vi "PSUChargeRelay.vi"(4 "PSU3 Control Panel":T1={"HV Off State"=FALSE, "HV On State"=FALSE, "HV Arm"=FALSE, "HV On"=FALSE, "Charge relay DIO"="DAQ0/port0/line3", "Dump relay DIO"="DAQ0/port0/line4", "HV Arm DIO"="DAQ0/port0/line5", "HV On DIO"="DAQ0/port0/line6", "Bank Voltage [kV]"={0.0, 0.0}, "Vdemand Counter"="Timing1/ctr1", "RevTach Calibration"=path "Z:/Data/Calibration/Reverse Tachometer/PSU2_RevTachCalibration.csv", "Vdemand"=FALSE, "Vmeasure Counter"="Timing1/ctr2", "Tach Calibration"=path "Z:/Data/Calibration/Tachometer/PSU2_TachCalibration.csv", "Vmeasure"=FALSE, "Vdemand [kV]"=0.0, "Charge Relay"=FALSE, "Dump Relay"=FALSE} {"Bank Voltage [kV]" scale=0.01..10.0 scale format="%#_3g"}, 6 "PSU2 Control Panel":T1 {"Bank Voltage [kV]" scale=0.01..10.0 scale format="%#_3g"}, 10 "PSU Relay Variant":T2, 11 "Experiment State in":T3 {"Global Settings"."Initial Background Values"."Cryo temp [K]" format="%#_4g"; "RIO Settings"."Card Settings"."Sample Rate" format="%#_3p"; "Timing Settings"."Timing Channel Settings"."FrontPanelTime" format="%.3p"; "Timing Settings"."Timing Channel Settings"."Pulse width (s)" format="%.3p"; "Timing Settings"."Timing Channel Settings"."Delay (s)" format="%.3p"; "DAQ Settings"."Card Settings"."Global Edge Type" items=["Rising"=10280, "Falling"=10171]; "DAQ Settings"."Card Settings"."Sample Rate" format="%#_3p"}) -> (3 "Experiment State out":T3 {"Global Settings"."Initial Background Values"."Cryo temp [K]" format="%#_4g"; "RIO Settings"."Card Settings"."Sample Rate" format="%#_3p"; "Timing Settings"."Timing Channel Settings"."FrontPanelTime" format="%.3p"; "Timing Settings"."Timing Channel Settings"."Pulse width (s)" format="%.3p"; "Timing Settings"."Timing Channel Settings"."Delay (s)" format="%.3p"; "DAQ Settings"."Card Settings"."Global Edge Type" items=["Rising"=10280, "Falling"=10171]; "DAQ Settings"."Card Settings"."Sample Rate" format="%#_3p"})   [LabVIEW 2014]
uses:
  Controls/PSUPanel-Arming.ctl
  Controls/ExperimentStateCluster.ctl
  Controls/DigitizerSettingsChannelSettings.ctl
  Controls/DigitizerSettingsCardSettingsArray.ctl
  Controls/DigitizerSettingsCardSettings.ctl
  Controls/TimingSettings.ctl
  Controls/TimingCardSettings.ctl
  Controls/TimingChannelSettings.ctl
  Controls/RIOSettingsExperimentStateCluster.ctl
  Controls/RIOChannelSettingsArrayExperimentStateCluster.ctl
  Controls/RIOSettingsChannelSettings.ctl
  Controls/RIOSettingsCardSettingsArray.ctl
  Controls/RIOSettingsCardSettings.ctl
  <vilib>/userdefined/High Color/nirio_resource_hc.ctl
  Controls/RIOData.ctl
  Controls/DIOChannel.ctl
  Controls/Global Settings/GlobalSettings.ctl
  Controls/Global Settings/InitialBackgroundValues.ctl
  Controls/Global Settings/GasPuffing.ctl
  Controls/Global Settings/PSUVoltages.ctl
  Controls/Global Settings/ScopeDetails.ctl
  Controls/Calibrations/Calibrations.ctl
  Controls/Calibrations/CryoTemoCalibration.ctl
  Controls/Calibrations/PSU2TachCalibration.ctl
  Controls/Calibrations/PSU3TachCalibration.ctl
  Controls/TachTasks.ctl
  Controls/PSU2TachometerControls.ctl
  Controls/PSU3TachometerControls.ctl
  Controls/PSU2DIOChannels.ctl
  Controls/PSU3DIOChannels.ctl
  Controls/PSU2ReverseTachometerControls.ctl
  Controls/PSU3ReverseTachometerControls.ctl
  Controls/PSUControlVariant.ctl
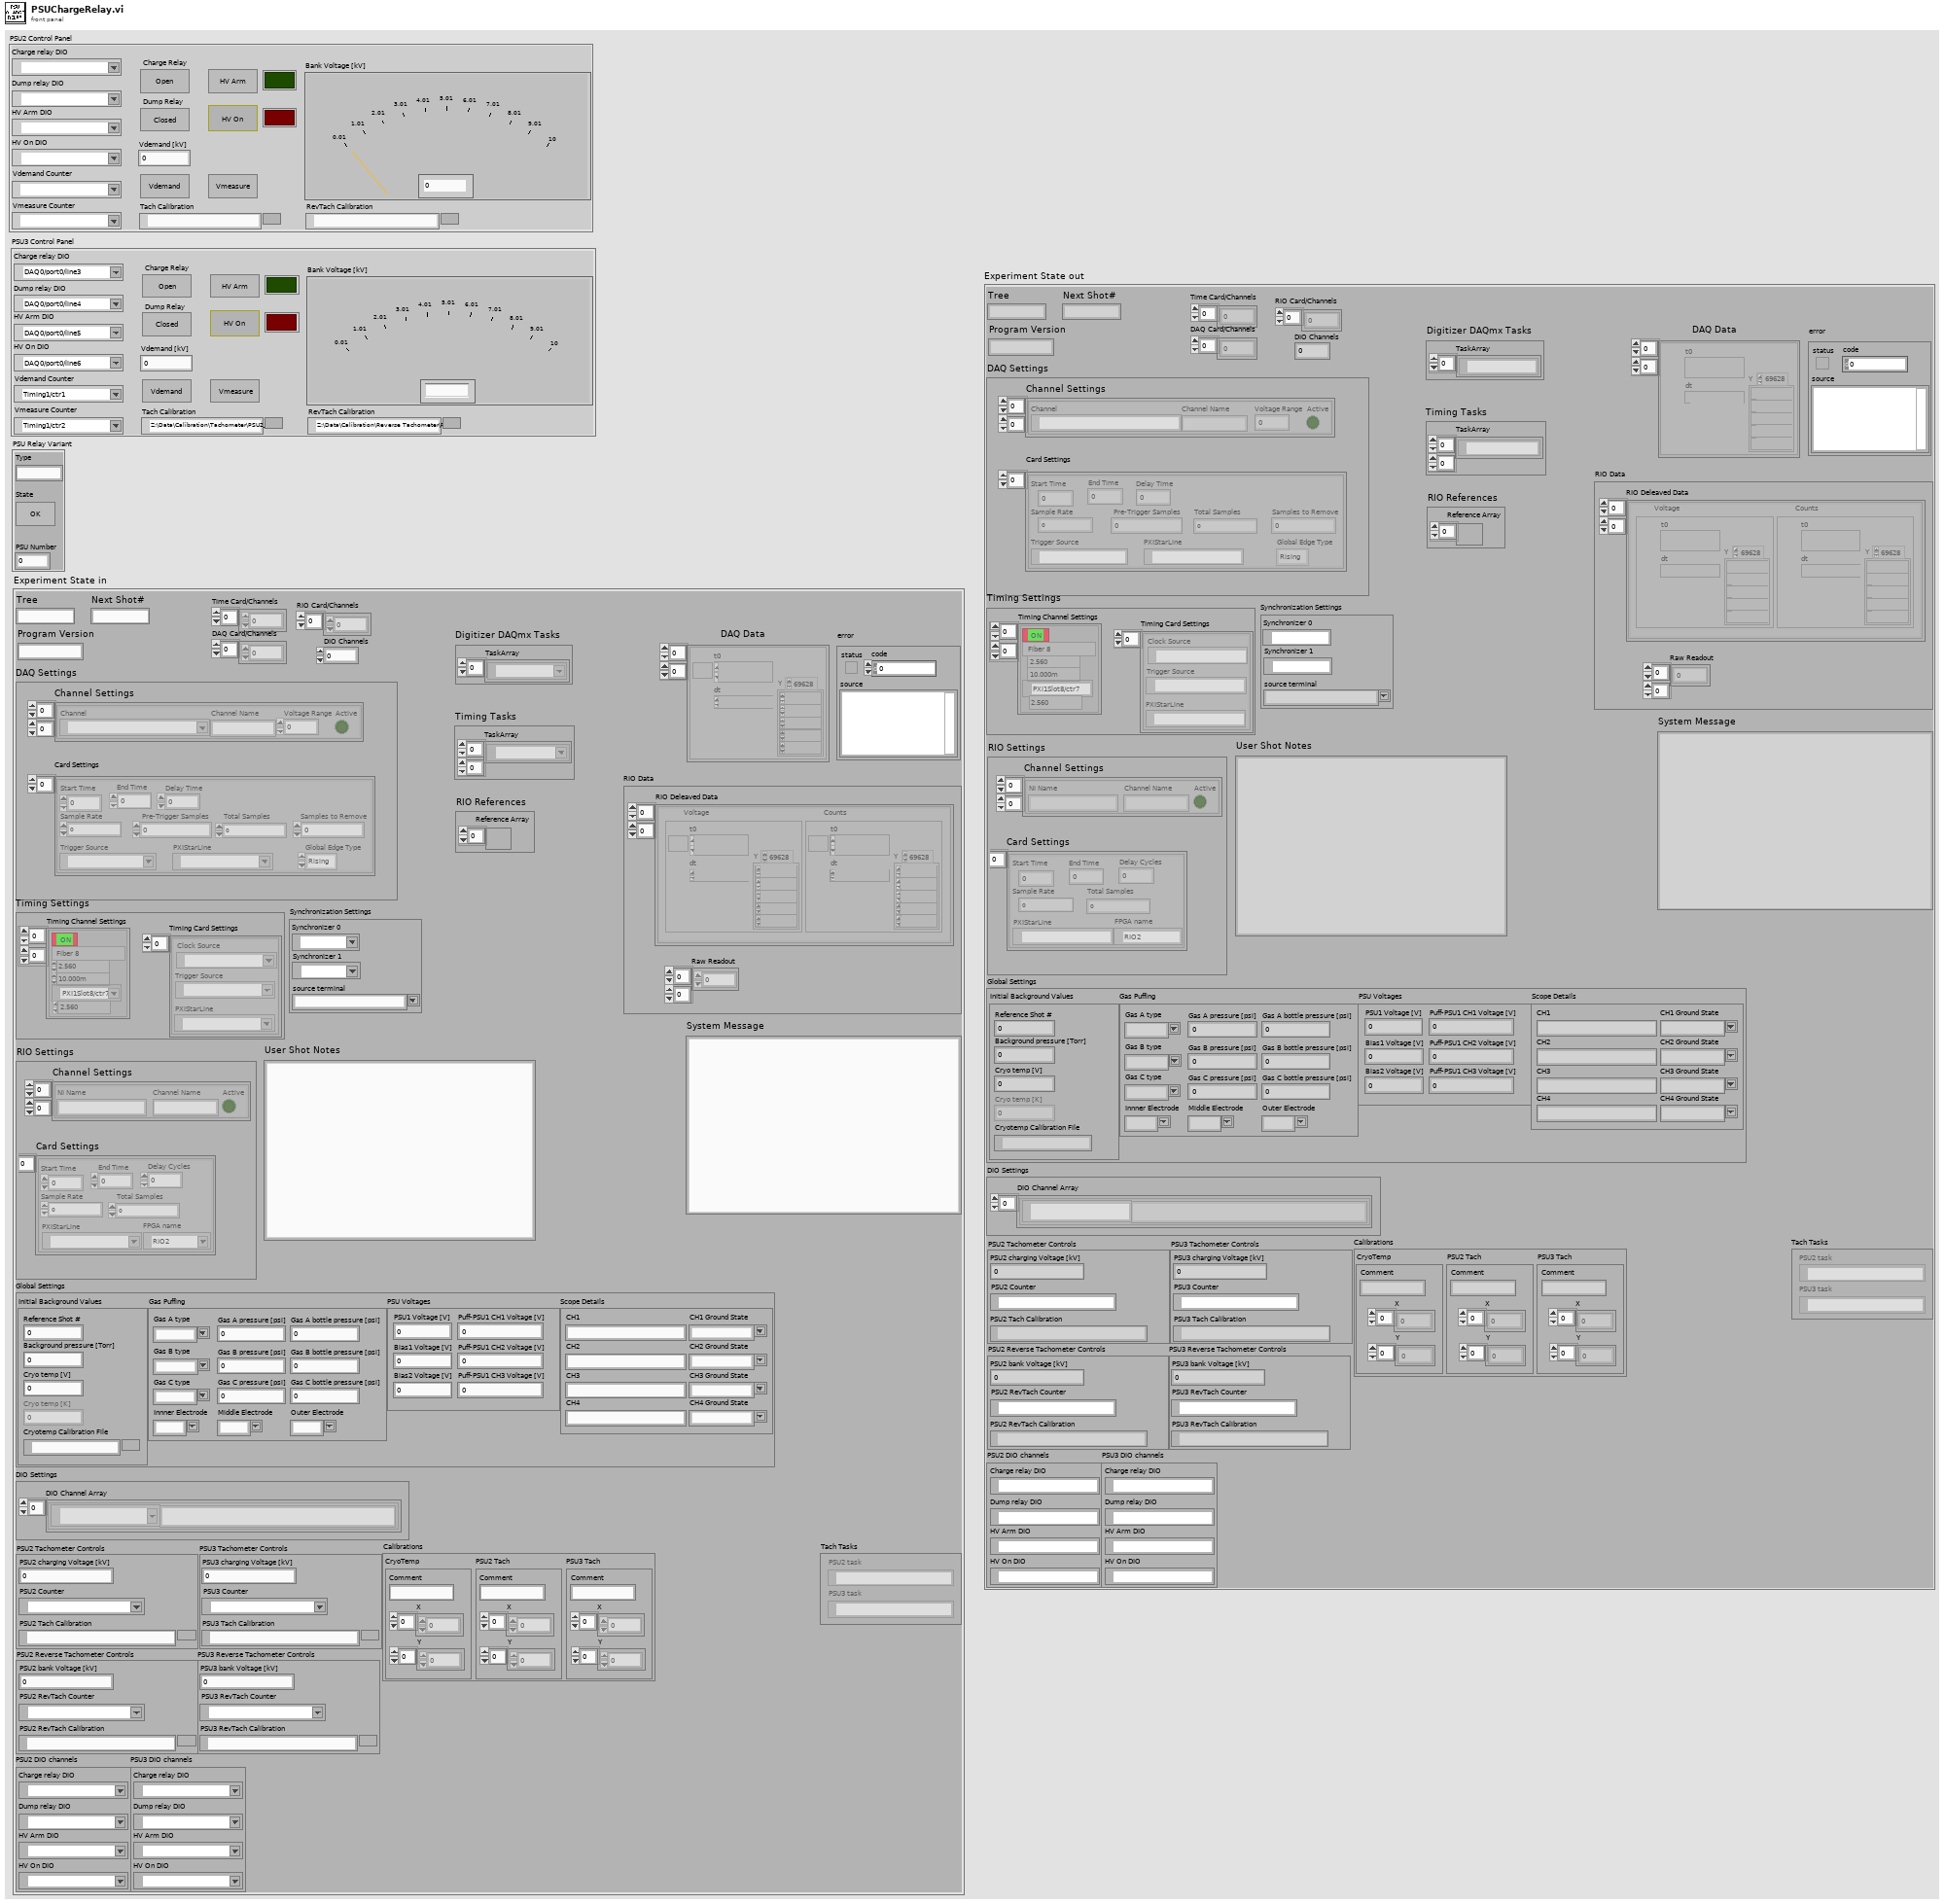
[diagram p1: front panel]
types:
  T1 = typedef "PSUPanel-Arming.ctl" = cluster{"HV Off State":bool, "HV On State":bool, "HV Arm":bool, "HV On":bool, "Charge relay DIO":tag, "Dump relay DIO":tag, "HV Arm DIO":tag, "HV On DIO":tag, "Bank Voltage [kV]":cluster{dbl, dbl}, "Vdemand Counter":tag, "RevTach Calibration":path, "Vdemand":bool, "Vmeasure Counter":tag, "Tach Calibration":path, "Vmeasure":bool, "Vdemand [kV]":dbl, "Charge Relay":bool, "Dump Relay":bool}
  T2 = typedef "PSUControlVariant.ctl" = cluster{"State":bool, "PSU Number":i32, "Type":string}
  T3 = typedef "ExperimentStateCluster.ctl" = cluster{"error":errorcluster, "Digitizer DAQmx Tasks":cluster{"TaskArray":refnum<k21>[]}, "DAQ Settings":cluster{"Channel Settings":T4[][], "Card Settings":T5}, "Synchronization Settings":cluster{"Synchronizer 0":refnum<k15>, "source terminal":string, "Synchronizer 1":refnum<k15>}, "DAQ Data":waveform(dbl)[][], "Next Shot#":string, "System Message":string, "User Shot Notes":string, "Timing Settings":T7, "Timing Tasks":cluster{"TaskArray":refnum<k21>[][]}, "Tree":string, "Time Card/Channels":i32[], "DAQ Card/Channels":i32[], "Program Version":string, "RIO Settings":T10, "RIO References":cluster{"Reference Array":refnum<k20>[]}, "RIO Data":T16, "RIO Card/Channels":i32[], "DIO Channels":i32, "DIO Settings":cluster{"DIO Channel Array":T17[]}, "Global Settings":T18, "Calibrations":T23, "Tach Tasks":T27, "PSU2 Tachometer Controls":T28, "PSU3 Tachometer Controls":T29, "PSU2 DIO channels":T30, "PSU3 DIO channels":T31, "PSU2 Reverse Tachometer Controls":T32, "PSU3 Reverse Tachometer Controls":T33}
  T4 = typedef "DigitizerSettingsChannelSettings.ctl" = cluster{"Channel":tag, "Channel Name":string, "Voltage Range":dbl, "Active":bool}
  T5 = typedef "DigitizerSettingsCardSettingsArray.ctl" = T6[]
  T6 = typedef "DigitizerSettingsCardSettings.ctl" = cluster{"Start Time":dbl, "End Time":dbl, "Sample Rate":dbl, " Pre-Trigger Samples":u32, "Total Samples":i32, "Samples to Remove":u32, "Trigger Source":tag, "Global Edge Type":i32, "PXIStarLine":tag, "Delay Time":dbl}
  T7 = typedef "TimingSettings.ctl" = cluster{"Timing Card Settings":T8[], "Timing Channel Settings":T9[][]}
  T8 = typedef "TimingCardSettings.ctl" = cluster{"Trigger Source":tag, "Clock Source":tag, "PXIStarLine":tag}
  T9 = typedef "TimingChannelSettings.ctl" = cluster{"Delay (s)":dbl, "Pulse width (s)":dbl, "Active":bool, "Channel Name":string, "counter":tag, "FrontPanelTime":dbl}
  T10 = typedef "RIOSettingsExperimentStateCluster.ctl" = cluster{"Channel Settings":T11, "Card Settings":T13}
  T11 = typedef "RIOChannelSettingsArrayExperimentStateCluster.ctl" = T12[][]
  T12 = typedef "RIOSettingsChannelSettings.ctl" = cluster{"Channel Name":string, "Active":bool, "NI Name":string}
  T13 = typedef "RIOSettingsCardSettingsArray.ctl" = T14[]
  T14 = typedef "RIOSettingsCardSettings.ctl" = cluster{"Start Time":dbl, "End Time":dbl, "Sample Rate":dbl, "Total Samples":u64, "PXIStarLine":tag, "Delay Cycles":u64, "FPGA name":T15}
  T15 = typedef "nirio_resource_hc.ctl" = tag
  T16 = typedef "RIOData.ctl" = cluster{"RIO Deleaved Data":cluster{"Voltage":waveform(dbl), "Counts":waveform(i16)}[][], "Raw Readout":u64[][]}
  T17 = typedef "DIOChannel.ctl" = cluster{"Channel Name":string, "NI Name":tag}
  T18 = typedef "GlobalSettings.ctl" = cluster{"Initial Background Values":T19, "Gas Puffing":T20, "PSU Voltages":T21, "Scope Details":T22}
  T19 = typedef "InitialBackgroundValues.ctl" = cluster{"Reference Shot #":dbl, "Background pressure [Torr]":dbl, "Cryo temp [V]":dbl, "Cryo temp [K]":dbl, "Cryotemp Calibration File":path}
  T20 = typedef "GasPuffing.ctl" = cluster{"Gas A type":string, "Gas B type":string, "Gas C type":string, "Gas A pressure [psi]":dbl, "Gas B pressure [psi]":dbl, "Gas C pressure [psi]":dbl, "Innner Electrode":string, "Middle Electrode":string, "Outer Electrode":string, "Gas A bottle pressure [psi]":dbl, "Gas B bottle pressure [psi]":dbl, "Gas C bottle pressure [psi]":dbl}
  T21 = typedef "PSUVoltages.ctl" = cluster{"Bias1 Voltage [V]":dbl, "Bias2 Voltage [V]":dbl, "PSU1 Voltage [V]":dbl, "Puff-PSU1 CH1 Voltage [V]":dbl, "Puff-PSU1 CH2 Voltage [V]":dbl, "Puff-PSU1 CH3 Voltage [V]":dbl}
  T22 = typedef "ScopeDetails.ctl" = cluster{"CH1":string, "CH2":string, "CH3":string, "CH4":string, "CH1 Ground State":string, "CH2 Ground State":string, "CH3 Ground State":string, "CH4 Ground State":string}
  T23 = typedef "Calibrations.ctl" = cluster{"CryoTemp":T24, "PSU2 Tach":T25, "PSU3 Tach":T26}
  T24 = typedef "CryoTemoCalibration.ctl" = cluster{"Comment":string, "X":dbl[], "Y":dbl[]}
  T25 = typedef "PSU2TachCalibration.ctl" = cluster{"Comment":string, "X":dbl[], "Y":dbl[]}
  T26 = typedef "PSU3TachCalibration.ctl" = cluster{"Comment":string, "X":dbl[], "Y":dbl[]}
  T27 = typedef "TachTasks.ctl" = cluster{"PSU2 task":refnum<k21>, "PSU3 task":refnum<k21>}
  T28 = typedef "PSU2TachometerControls.ctl" = cluster{"PSU2 Tach Calibration":path, "PSU2 charging Voltage [kV]":dbl, "PSU2 Counter":tag}
  T29 = typedef "PSU3TachometerControls.ctl" = cluster{"PSU3 Tach Calibration":path, "PSU3 charging Voltage [kV]":dbl, "PSU3 Counter":tag}
  T30 = typedef "PSU2DIOChannels.ctl" = cluster{"Charge relay DIO":tag, "Dump relay DIO":tag, "HV Arm DIO":tag, "HV On DIO":tag}
  T31 = typedef "PSU3DIOChannels.ctl" = cluster{"Charge relay DIO":tag, "Dump relay DIO":tag, "HV Arm DIO":tag, "HV On DIO":tag}
  T32 = typedef "PSU2ReverseTachometerControls.ctl" = cluster{"PSU2 RevTach Calibration":path, "PSU2 bank Voltage [kV]":dbl, "PSU2 RevTach Counter":tag}
  T33 = typedef "PSU3ReverseTachometerControls.ctl" = cluster{"PSU3 RevTach Calibration":path, "PSU3 bank Voltage [kV]":dbl, "PSU3 RevTach Counter":tag}
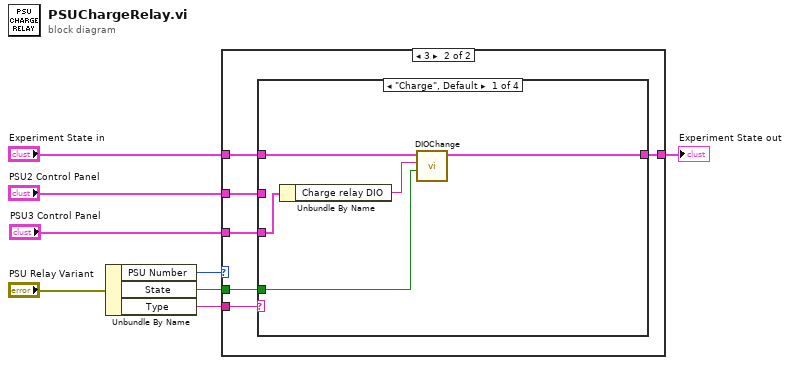
[diagram p0: block diagram]
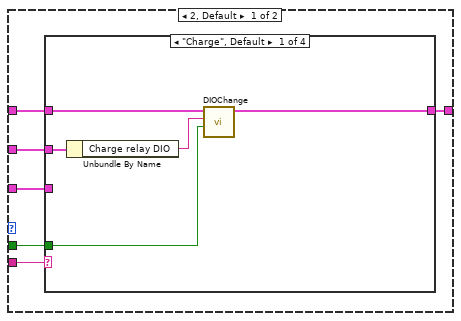
[diagram p2: hidden frame]
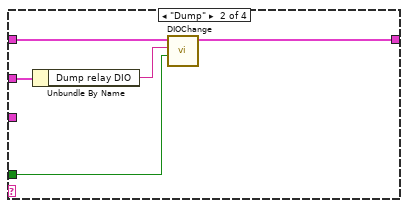
[diagram p3: hidden frame]
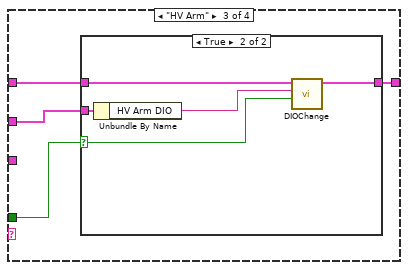
[diagram p4: hidden frame]
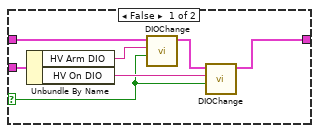
[diagram p5: hidden frame]
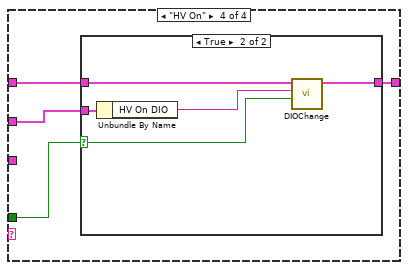
[diagram p6: hidden frame]
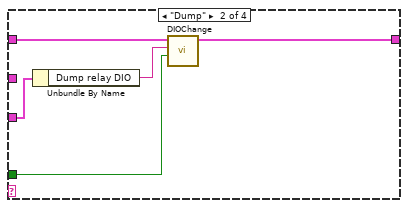
[diagram p8: hidden frame]
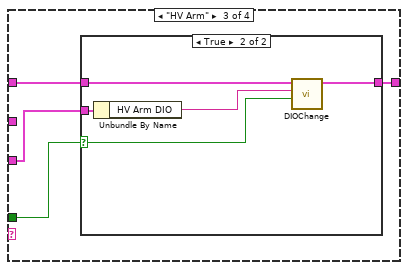
[diagram p9: hidden frame]
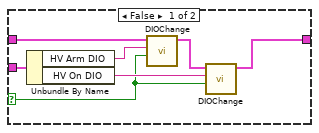
[diagram p10: hidden frame]
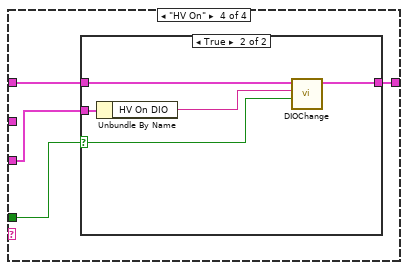
[diagram p11: hidden frame]
diagram:
  n1 = Unbundle By Name("PSU Relay Variant") -> ("PSU Number"=w3:i32, "State"=w5:bool, "Type"=w1:string)
  n2 = case shown="3" w3 {
    tunnel: "PSU2 Control Panel" -> [w14 w56]
    tunnel: [w13 w55] -> w7
    tunnel: "Experiment State in" -> [w12 w54]
    tunnel: w5 -> [w11 w53]
    tunnel: "PSU3 Control Panel" -> [w10 w52]
    tunnel: w1 -> [w9 w51]
    frame 2, Default {
      n3 = case shown="\"Charge\", Default" w9 {
        tunnel: w14 -> [w19 w24 w28 w44]
        tunnel: [w18 w23 w27 w43] -> w13
        tunnel: w12 -> [w17 w22 w25 w41]
        tunnel: w11 -> [w16 w21 w26 w42]
        tunnel: w10 -> [_ _ _ _]
        frame "Charge", Default {
          n4 = Unbundle By Name(w19) -> ("Charge relay DIO"=w15:tag)
          n5 = call "DIOChange.vi"("Relay State"=w16, "Charge relay DIO"=w15, "Experiment State in"=w17) -> ("Experiment State out"=w18:T3)  [unwired: 8 in]
        }
        frame "Dump" {
          n6 = Unbundle By Name(w24) -> ("Dump relay DIO"=w20:tag)
          n7 = call "DIOChange.vi"("Relay State"=w21, "Charge relay DIO"=w20, "Experiment State in"=w22) -> ("Experiment State out"=w23:T3)  [unwired: 8 in]
        }
        frame "HV Arm" {
          n8 = case shown="True" w26 {
            selector: w26 -> [w30 w37]
            tunnel: w28 -> [w35 w40]
            tunnel: [w32 w39] -> w27
            tunnel: w25 -> [w29 w36]
            frame False {
              n9 = Unbundle By Name(w35) -> ("HV Arm DIO"=w34:tag, "HV On DIO"=w31:tag)
              n10 = call "DIOChange.vi"("Relay State"=w30, "Charge relay DIO"=w34, "Experiment State in"=w29) -> ("Experiment State out"=w33:T3)  [unwired: 8 in]
              n11 = call "DIOChange.vi"("Relay State"=w30, "Charge relay DIO"=w31, "Experiment State in"=w33) -> ("Experiment State out"=w32:T3)  [unwired: 8 in]
            }
            frame True {
              n12 = Unbundle By Name(w40) -> ("HV Arm DIO"=w38:tag)
              n13 = call "DIOChange.vi"("Relay State"=w37, "Charge relay DIO"=w38, "Experiment State in"=w36) -> ("Experiment State out"=w39:T3)  [unwired: 8 in]
            }
          }
        }
        frame "HV On" {
          n14 = case shown="True" w42 {
            selector: w42 -> [_ w47]
            tunnel: w44 -> [_ w50]
            tunnel: [w45 w49] -> w43
            tunnel: w41 -> [w45 w46]
            frame False {
            }
            frame True {
              n15 = Unbundle By Name(w50) -> ("HV On DIO"=w48:tag)
              n16 = call "DIOChange.vi"("Relay State"=w47, "Charge relay DIO"=w48, "Experiment State in"=w46) -> ("Experiment State out"=w49:T3)  [unwired: 8 in]
            }
          }
        }
      }
    }
    frame 3 {
      n17 = case shown="\"Charge\", Default" w51 {
        tunnel: w56 -> [_ _ _ _]
        tunnel: [w61 w66 w70 w86] -> w55
        tunnel: w54 -> [w60 w65 w68 w84]
        tunnel: w53 -> [w59 w64 w69 w85]
        tunnel: w52 -> [w57 w62 w67 w83]
        frame "Charge", Default {
          n18 = Unbundle By Name(w57) -> ("Charge relay DIO"=w58:tag)
          n19 = call "DIOChange.vi"("Relay State"=w59, "Charge relay DIO"=w58, "Experiment State in"=w60) -> ("Experiment State out"=w61:T3)  [unwired: 8 in]
        }
        frame "Dump" {
          n20 = Unbundle By Name(w62) -> ("Dump relay DIO"=w63:tag)
          n21 = call "DIOChange.vi"("Relay State"=w64, "Charge relay DIO"=w63, "Experiment State in"=w65) -> ("Experiment State out"=w66:T3)  [unwired: 8 in]
        }
        frame "HV Arm" {
          n22 = case shown="True" w69 {
            selector: w69 -> [w72 w79]
            tunnel: w67 -> [w77 w82]
            tunnel: [w74 w81] -> w70
            tunnel: w68 -> [w71 w78]
            frame False {
              n23 = Unbundle By Name(w77) -> ("HV Arm DIO"=w76:tag, "HV On DIO"=w73:tag)
              n24 = call "DIOChange.vi"("Relay State"=w72, "Charge relay DIO"=w76, "Experiment State in"=w71) -> ("Experiment State out"=w75:T3)  [unwired: 8 in]
              n25 = call "DIOChange.vi"("Relay State"=w72, "Charge relay DIO"=w73, "Experiment State in"=w75) -> ("Experiment State out"=w74:T3)  [unwired: 8 in]
            }
            frame True {
              n26 = Unbundle By Name(w82) -> ("HV Arm DIO"=w80:tag)
              n27 = call "DIOChange.vi"("Relay State"=w79, "Charge relay DIO"=w80, "Experiment State in"=w78) -> ("Experiment State out"=w81:T3)  [unwired: 8 in]
            }
          }
        }
        frame "HV On" {
          n28 = case shown="True" w85 {
            selector: w85 -> [_ w89]
            tunnel: w83 -> [_ w92]
            tunnel: [w87 w91] -> w86
            tunnel: w84 -> [w87 w88]
            frame False {
            }
            frame True {
              n29 = Unbundle By Name(w92) -> ("HV On DIO"=w90:tag)
              n30 = call "DIOChange.vi"("Relay State"=w89, "Charge relay DIO"=w90, "Experiment State in"=w88) -> ("Experiment State out"=w91:T3)  [unwired: 8 in]
            }
          }
        }
      }
    }
  }
  "Experiment State out" <- w7
